vi "1.vi"() -> ()   [LabVIEW 2015]
uses:
  Global 2.vi
panel:
  out "Waveform Chart 2":dbl(graph)
  out "Waveform Chart":dbl(graph)
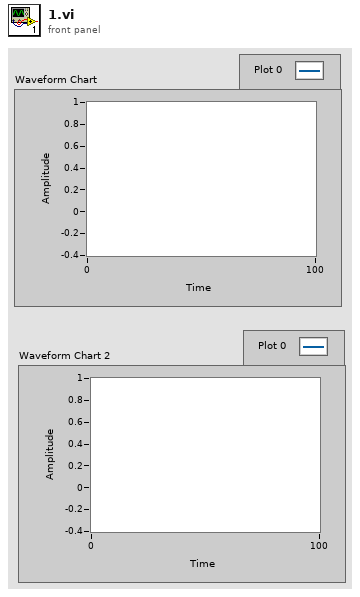
[diagram p1: front panel]
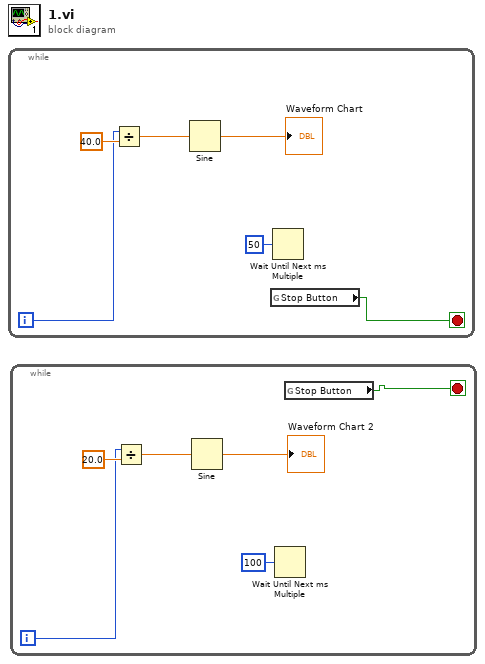
[diagram p0: block diagram]
diagram:
  n1 = while {
    i -> [w5]
    stop <- w1 stop-if-true
    n2 = Divide(x=w5, y=40.0) -> (x/y=w4:dbl)
    n3 = Sine(x=w4) -> (sin(x)=→"Waveform Chart":dbl)
    n4 = global read "Global 2.vi" "Stop Button"() -> (w1:bool)
    n5 = Wait Until Next ms Multiple(millisecond multiple=u32 50) -> ()  [unwired: 1 out]
  }
  n6 = while {
    i -> [w11]
    stop <- w7 stop-if-true
    n7 = Divide(x=w11, y=20.0) -> (x/y=w10:dbl)
    n8 = Sine(x=w10) -> (sin(x)=→"Waveform Chart 2":dbl)
    n9 = Wait Until Next ms Multiple(millisecond multiple=u32 100) -> ()  [unwired: 1 out]
    n10 = global read "Global 2.vi" "Stop Button"() -> (w7:bool)
  }
